vi "Test_DO.vi"() -> ()   [LabVIEW 2023]
uses:
  DI_DO/DI_DO.lvclass
panel:
  out "STATUS":string
  out "error out":errorcluster
  out "Error":string
  in  "DO":bool
  in  "PIN":i8
  in  "Input":T1
  in  "error in (no error)":errorcluster
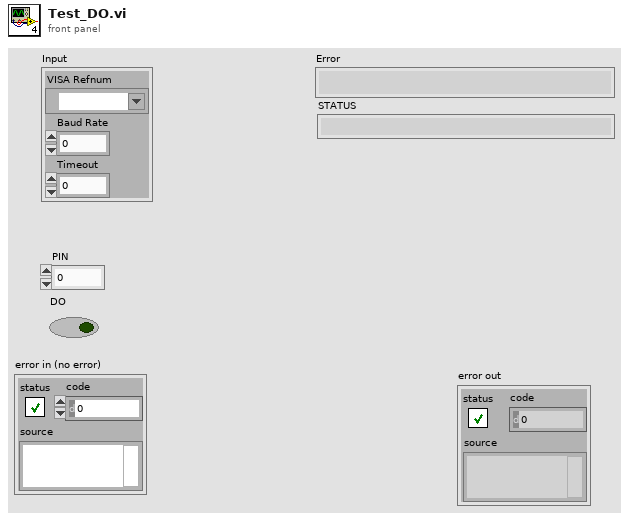
[diagram p1: front panel]
types:
  T1 = cluster{"VISA Refnum":refnum<visa-resource-name>, "Baud Rate":u32, "Timeout":u32}
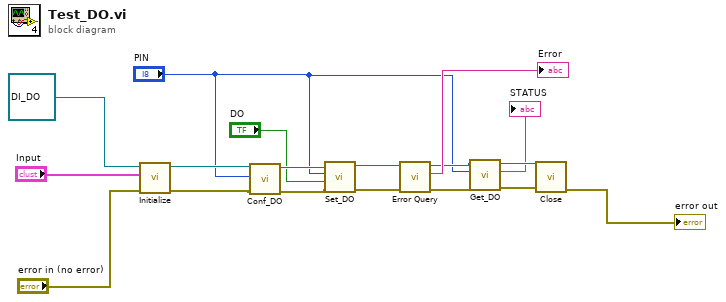
[diagram p0: block diagram]
diagram:
  n1 = call-dynamic "Initialize.vi"("error in (no error)"="error in (no error)", "Input"="Input", "Driver in"=refnum<class "DI_DO.lvclass"> refnum ("Driver_DI_DO.lvlib:DI_DO.lvclass")) -> ("error out"=w16:errorcluster, "Driver out"=w15:refnum<class "DI_DO.lvclass">)  [unwired: 7 in]
  n2 = call-dynamic "Conf_DO.vi"("error in (no error)"=w16, "PIN Number"="PIN", "DI_DO in"=w15) -> ("error out"=w13:errorcluster, "DI_DO out"=w12:refnum<class "DI_DO.lvclass">)  [unwired: 7 in]
  n3 = call-dynamic "Set_DO.vi"("error in (no error)"=w13, "DO"="DO", "PIN"="PIN", "DI_DO in"=w12) -> ("error out"=w10:errorcluster, "DI_DO out"=w9:refnum<class "DI_DO.lvclass">)  [unwired: 6 in]
  n4 = call-dynamic "Error Query.vi"("error in (no error)"=w10, "Driver in"=w9) -> ("error out"=w7:errorcluster, "read buffer"=→"Error":string, "Driver out"=w6:refnum<class "DI_DO.lvclass">)  [unwired: 7 in]
  n5 = call-dynamic "Get_DO.vi"("error in (no error)"=w7, "PIN Number"="PIN", "DI_DO in"=w6) -> ("error out"=w5:errorcluster, "STATUS"=→"STATUS":string, "DI_DO out"=w4:refnum<class "DI_DO.lvclass">)  [unwired: 6 in]
  n6 = call-dynamic "Close.vi"("error in (no error)"=w5, "Driver in"=w4) -> ("error out"=→"error out":errorcluster)  [unwired: 8 in, 1 out]
